vi "ackCommand.vi"(4 "ack":i32, 6 "result":string, 7 "CommandValue":T1, 8 "error in (no error)":errorcluster, 9 "error":i32, 10 "cmdSeqNum":i32, 11 "SALCommunicatorController in":refnum<class "SALCommunicatorController.lvclass">) -> (0 "error out":errorcluster, 3 "SALCommunicatorController out":refnum<class "SALCommunicatorController.lvclass">)   [LabVIEW 2016, in "SALCommunicatorController.lvclass"]
uses:
  SALCommunicatorController.lvclass
  Typedefs/CommandValue.ctl
  ts_sallv_exa/DataTypes/ackcmd.ctl
  ts_sallv_exa/SALLV_EXA.lvlib
  Typedefs/EXATypedefs.lvlib
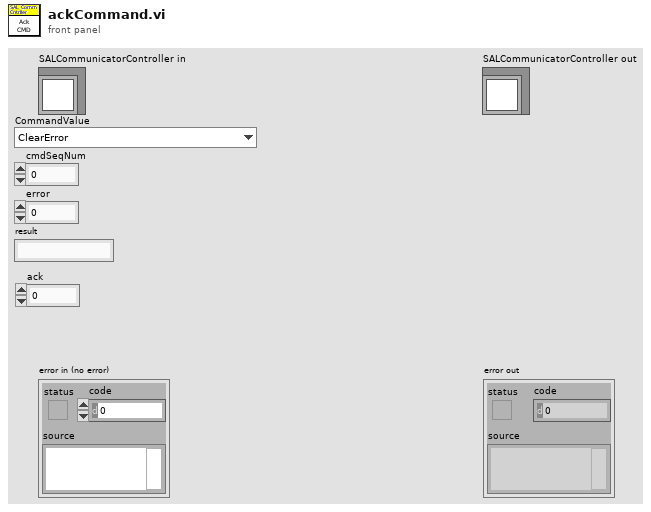
[diagram p1: front panel]
types:
  T1 = typedef "EXATypedefs.lvlib/CommandValue.ctl" = enum16{"ClearError", "Disable", "Enable", "Exit", "GoToStandby", "OnHeartbeat", "OnIncomingMessagingError", "OnInterrupt", "Start"}
  T2 = typedef "SALLV_EXA.lvlib/ackcmd.ctl" = cluster{"cmdSeqNum":i32, "ack":i32, "error":i32, "result":string}
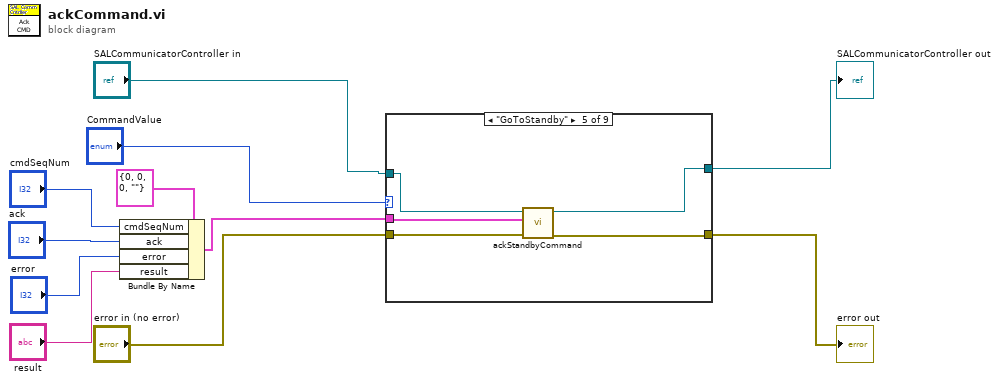
[diagram p0: block diagram]
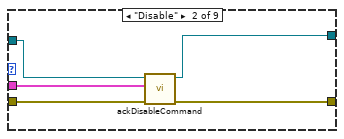
[diagram p3: hidden frame]
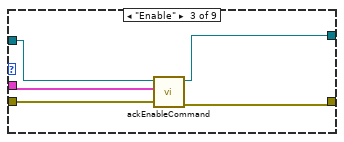
[diagram p4: hidden frame]
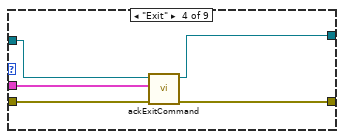
[diagram p5: hidden frame]
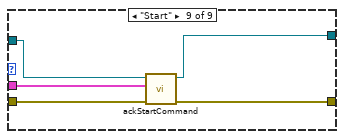
[diagram p9: hidden frame]
diagram:
  n1 = Bundle By Name(cluster=T2 {"cmdSeqNum"=0, "ack"=0, "error"=0, "result"=""} ("ackcmd_Ctl"), "cmdSeqNum"="cmdSeqNum", "ack"="ack", "error"="error", "result"="result") -> (w7:T2)
  n2 = case shown="\"GoToStandby\"" "CommandValue" {
    tunnel: "error in (no error)" -> [w13 w18 w23 w28 w33 w35 w37 w39 w44]
    tunnel: [w13 w17 w22 w27 w32 w35 w37 w39 w43] -> w10
    tunnel: w7 -> [_ w16 w21 w26 w31 _ _ _ w42]
    tunnel: "SALCommunicatorController in" -> [w12 w15 w19 w25 w30 w34 w36 w38 w41]
    tunnel: [w12 w14 w20 w24 w29 w34 w36 w38 w40] -> w1
    frame "ClearError", Default {
    }
    frame "Disable" {
      n3 = call "ackDisableCommand.vi"("error in (no error)"=w18, "ackcmd_Ctl"=w16, "SALCommunicatorController in"=w15) -> ("error out"=w17:errorcluster, "SALCommunicatorController out"=w14:refnum<class "SALCommunicatorController.lvclass">)  [unwired: 6 in, 1 out]
    }
    frame "Enable" {
      n4 = call "ackEnableCommand.vi"("error in (no error)"=w23, "ackcmd_Ctl"=w21, "SALCommunicatorController in"=w19) -> ("error out"=w22:errorcluster, "SALCommunicatorController out"=w20:refnum<class "SALCommunicatorController.lvclass">)  [unwired: 6 in, 1 out]
    }
    frame "Exit" {
      n5 = call "ackExitCommand.vi"("error in (no error)"=w28, "ackcmd_Ctl"=w26, "SALCommunicatorController in"=w25) -> ("error out"=w27:errorcluster, "SALCommunicatorController out"=w24:refnum<class "SALCommunicatorController.lvclass">)  [unwired: 6 in, 1 out]
    }
    frame "GoToStandby" {
      n6 = call "ackStandbyCommand.vi"("error in (no error)"=w33, "ackcmd_Ctl"=w31, "SALCommunicatorController in"=w30) -> ("error out"=w32:errorcluster, "SALCommunicatorController out"=w29:refnum<class "SALCommunicatorController.lvclass">)  [unwired: 6 in, 1 out]
    }
    frame "OnHeartbeat" {
    }
    frame "OnIncomingMessagingError" {
    }
    frame "OnInterrupt" {
    }
    frame "Start" {
      n7 = call "ackStartCommand.vi"("error in (no error)"=w44, "ackcmd_Ctl"=w42, "SALCommunicatorController in"=w41) -> ("error out"=w43:errorcluster, "SALCommunicatorController out"=w40:refnum<class "SALCommunicatorController.lvclass">)  [unwired: 6 in, 1 out]
    }
  }
  "error out" <- w10
  "SALCommunicatorController out" <- w1
